vi "Prepare Cluster.vi"(8 "Error In":errorcluster, 11 "Default Cluster":variant) -> (0 "Error Out":errorcluster, 2 "Name":string)   [LabVIEW 2016, in "Configit.lvlib"]
uses:
  Configit.lvlib
  <vilib>/Utility/VariantDataType/Type.ctl
  <vilib>/Waveform/DTblOps.llb/DTbl Empty Digital.vi
  <vilib>/Waveform/DWDTOps.llb/DWDT Empty Digital.vi
  <vilib>/Utility/VariantDataType/VariantType.lvlib
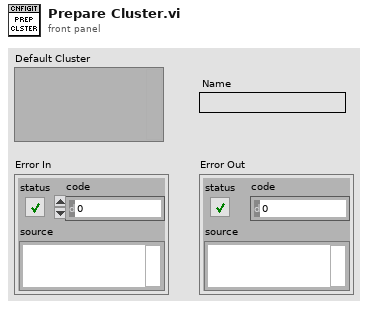
[diagram p1: front panel]
types:
  T1 = typedef "VariantType.lvlib/Type.ctl" = enum8{"Invalid Type", "Void", "I8", "I16", "I32", "I64", "U8", "U16", "U32", "U64", "Single Float", "Double Float", "Extended Float", "Single Complex", "Double Complex", "Extended Complex", "Enum U8", "Enum U16", "Enum U32", "Enum U64", "Single Float With Unit", "Double Float With Unit", "Extended Float With Unit", "Single Complex with Unit", "Double Complex with Unit", "Extended Complex with Unit", "Boolean", "String", "Path", "Picture", "Tag", "Array", "Cluster", "Variant", "LV Variant", "Waveform", "Timestamp", "Digital Waveform", "Digital Data", "ExpressData", "Refnum", "External Data", "VI", "Poly VI", "LabVIEW Class Instance", "Fixed Point"}
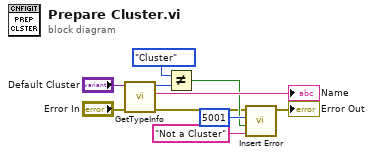
[diagram p0: block diagram]
diagram:
  n1 = call "GetTypeInfo.vi"("Error In"="Error In", "Variant"="Default Cluster") -> ("Error Out"=w4:errorcluster, "Name"=→"Name":string, "Type Enum"=w2:T1)  [unwired: 6 in, 1 out]
  n2 = Not Equal?(x=Type."Cluster", y=w2) -> (x != y?=w5:bool)
  n3 = call "Insert Error.vi"("Message"="Not a Cluster", "Insert (T)"=w5, "Code (5000)"=5001, "Error In"=w4) -> ("Error Out"=→"Error Out":errorcluster)  [unwired: 7 in]
